vi "ExReadGenericFile.vi"() -> ()   [LabVIEW 2010]
panel:
  in  "Data Type":T1(ring)
  in  "Full File Name":path
  in  "Swap Bytes":bool
  in  "Header Size (Bytes)":u32
  in  "Z Dimension( Number of Frames)":u32=1
  in  "Y Dimension":u32
  in  "X Dimension":u32
  in  "?":bool
  out "error out":errorcluster
  in  "error in (no error)":errorcluster
  # "ExReadGenericFile.vi\nThis VI will allow the user to read and display an image from a generic data file in which a header of known size is followed by one or more images of the same size.  The user must know the size of the header in bytes, the X/Y dimensions of an image, the number of images, the type of data and if byte swapping is required.\nWhen using this VI, be sure to hit the CLOSE IMAGE button when finished viewing the image.  This allows the image to be closed and the memory deallocated properly."
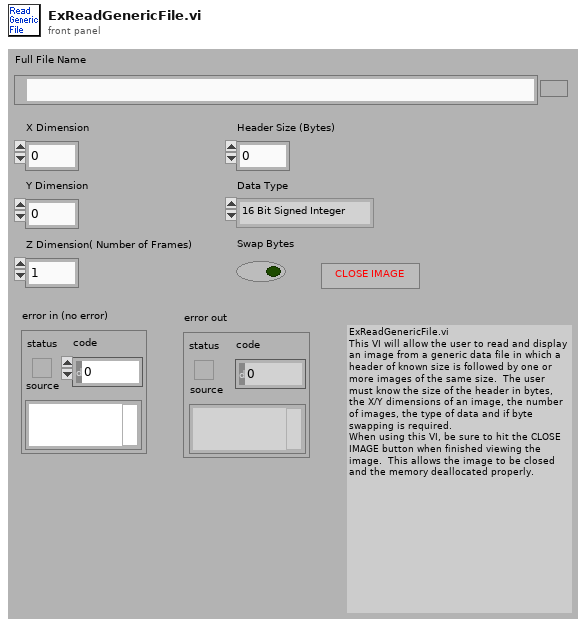
[diagram p1: front panel]
types:
  T1 = enum16{"16 Bit Signed Integer", "16 Bit Unsigned Integer", "32 Bit Signed Integer", "32 Bit Unsigned Integer", "8 Bit Signed Integer", "8 Bit Unsigned Integer", "32 Bit Floating Point", "64 Bit Floating Point"}
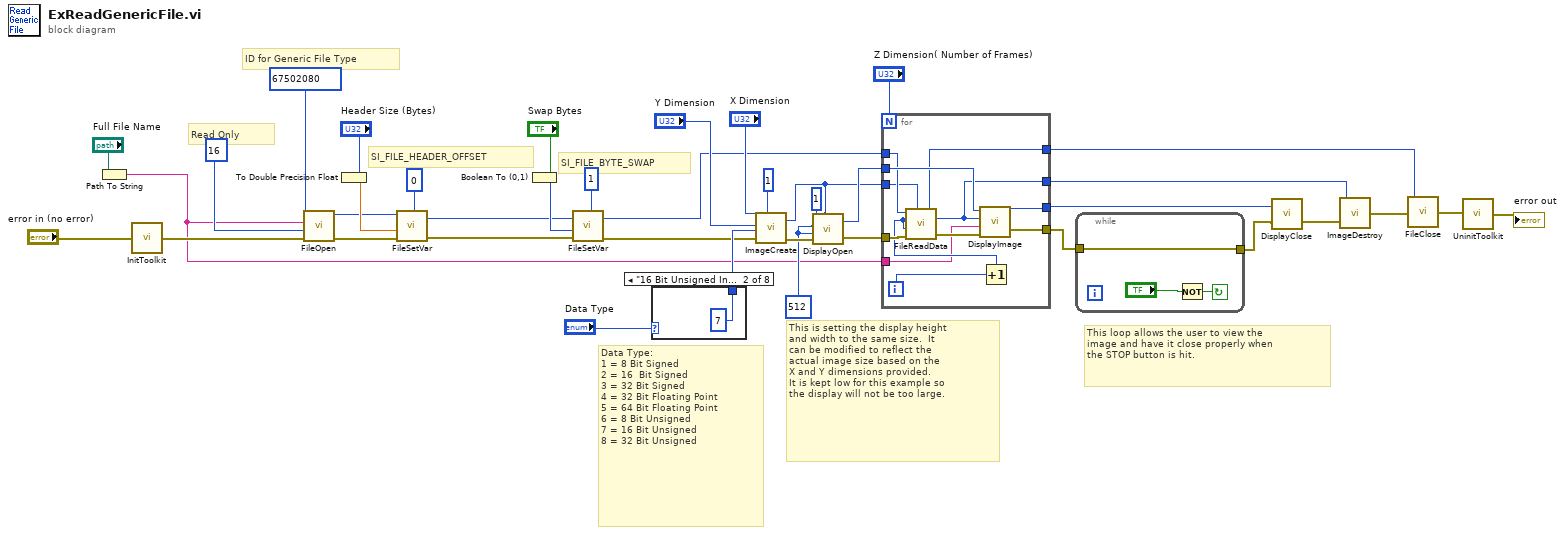
[diagram p0: block diagram]
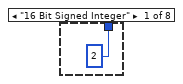
[diagram p2: hidden frame]
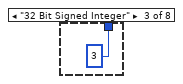
[diagram p3: hidden frame]
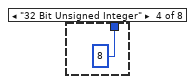
[diagram p4: hidden frame]
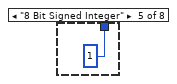
[diagram p5: hidden frame]
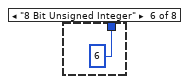
[diagram p6: hidden frame]
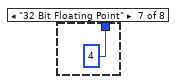
[diagram p7: hidden frame]
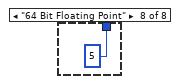
[diagram p8: hidden frame]
diagram:
  w36 = 512
  # "This loop allows the user to view the \nimage and have it close properly when\nthe STOP button is hit."
  # "This is setting the display height \nand width to the same size.  It \ncan be modified to reflect the\nactual image size based on the\nX and Y dimensions provided.\nIt is kept low for this example so\nthe display will not be too large."
  # "Data Type:\n1 = 8 Bit Signed\n2 = 16  Bit Signed\n3 = 32 Bit Signed\n4 = 32 Bit Floating Point\n5 = 64 Bit Floating Point\n6 = 8 Bit Unsigned\n7 = 16 Bit Unsigned\n8 = 32 Bit Unsigned"
  # "SI_FILE_BYTE_SWAP"
  # "SI_FILE_HEADER_OFFSET"
  # "ID for Generic File Type"
  # "Read Only"
  n1 = Path To String(path="Full File Name") -> (string=w16:string)
  n2 = call <userlib>:"InitToolkit.vi"("error in"="error in (no error)") -> ("error out"=w39:errorcluster)
  n3 = call <userlib>:"FileOpen.vi"("error in"=w39, "File Operations"=16, "FileName"=w16, "File Type"=67502080) -> ("error out"=w15:errorcluster, "File Handle"=w4:u32)
  n4 = To Double Precision Float(number="Header Size (Bytes)") -> (double precision float=w10:dbl)
  n5 = call <userlib>:"FileSetVar.vi"("error in"=w15, "Value"=w10, "Parameter ID"=0, "File Handle"=w4) -> ("error out"=w14:errorcluster, "File Handle"=w2:u32)
  n6 = Boolean To (0,1)(Boolean="Swap Bytes") -> (0, 1=w8:i16)
  n7 = call <userlib>:"FileSetVar.vi"("error in"=w14, "Value"=w8, "Parameter ID"=1, "File Handle"=w2) -> ("error out"=w13:errorcluster, "File Handle"=w12:u32)
  n8 = case shown="\"16 Bit Unsigned Integer\"" "Data Type" {
    tunnel: [2 7 3 8 1 6 4 5] -> w17
    frame "16 Bit Signed Integer" {
    }
    frame "16 Bit Unsigned Integer" {
    }
    frame "32 Bit Signed Integer" {
    }
    frame "32 Bit Unsigned Integer" {
    }
    frame "8 Bit Signed Integer" {
    }
    frame "8 Bit Unsigned Integer" {
    }
    frame "32 Bit Floating Point" {
    }
    frame "64 Bit Floating Point" {
    }
  }
  n9 = call <userlib>:"ImageCreate.vi"("X dimension"="X Dimension", "Y dimension"="Y Dimension", "Data Type"=w17, "error in"=w13, "Number Of Frames"=1) -> ("Image Handle"=w32:u32, "error out"=w37:errorcluster)
  n10 = call <userlib>:"DisplayOpen.vi"("Image Handle"=w32, "error in"=w37, "Display Height"=w36, "Display Width"=w36, "Display Type"=1) -> ("error out"=w34:errorcluster, "Display Handle"=w33:u32)  [unwired: 1 in]
  n11 = for {
    N: "Z Dimension( Number of Frames)" -> [_]
    tunnel: w34 -> [w59]
    tunnel: w33 -> [w57]
    tunnel: w12 -> [w56]
    tunnel: w32 -> [w55]
    tunnel: [w52] -> w23
    tunnel: [w51] -> w31
    tunnel: [w50] -> w30
    tunnel: [w49] -> w27
    tunnel: w16 -> [w48]
    i -> [w54]
    n12 = Increment(x=w54) -> (x+1=w53:i32)
    n13 = call <userlib>:"FileReadData.vi"("File Handle"=w56, "Start Frame"=w53, "End Frame"=w53, "error in"=w59, "Image Handle"=w55) -> ("File Handle"=w50:u32, "Image Handle"=w49:u32, "error out"=w58:errorcluster)
    n14 = call <userlib>:"DisplayImage.vi"("error in"=w58, "Title"=w48, "Image Handle"=w49, "Display Handle"=w57) -> ("error out"=w52:errorcluster, "Display Handle"=w51:u32)
  }
  n15 = while {
    tunnel: w23 -> [w62]
    tunnel: [w62] -> w24
    stop <- w60 continue-if-true
    n16 = Not(x="?") -> (.not. x?=w60:bool)
  }
  n17 = call <userlib>:"DisplayClose.vi"("error in"=w24, "Display Handle"=w31) -> ("error out"=w29:errorcluster)
  n18 = call <userlib>:"ImageDestroy.vi"("error in"=w29, "Data handle"=w27) -> ("error out"=w28:errorcluster)
  n19 = call <userlib>:"FileClose.vi"("error in"=w28, "File Handle"=w30) -> ("error out"=w26:errorcluster)
  n20 = call <userlib>:"UninitToolkit.vi"("error in"=w26) -> ("error out"=→"error out":errorcluster)
